vi "Read Version.vi"(8 "error in (no error)":errorcluster, 11 "Engine in":refnum<class "Engine.lvclass">) -> (0 "error out":errorcluster, 2 "Version":string, 3 "Engine out":refnum<class "Engine.lvclass">)   [LabVIEW 2023, in "Engine.lvlib" / "Engine.lvclass"]
uses:
  Library/Engine.lvclass
  Library/Engine.lvclass/Engine.ctl
  <vilib>/Utility/LVLibp/NI_PackedLibraryUtility.lvlib
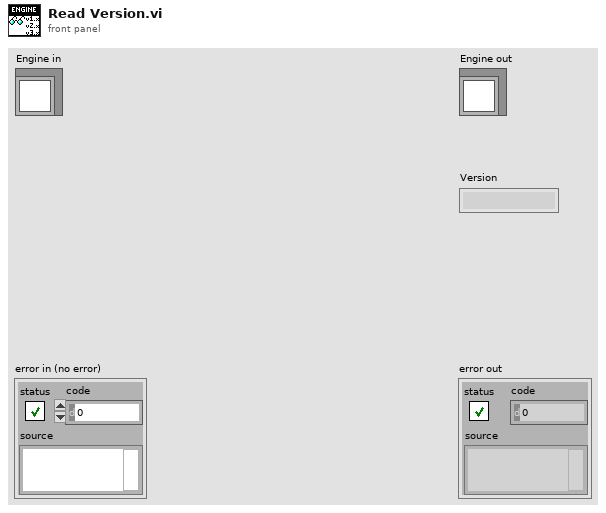
[diagram p1: front panel]
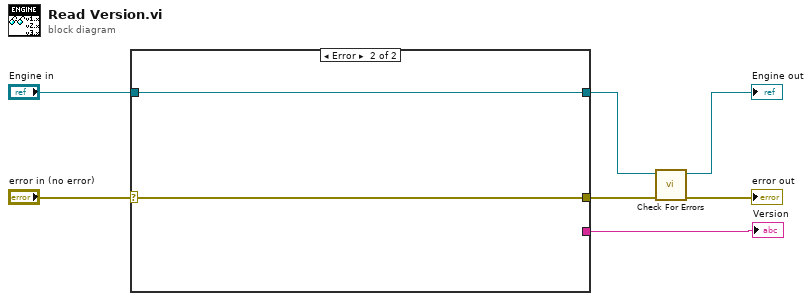
[diagram p0: block diagram]
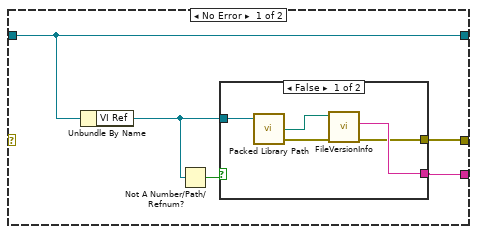
[diagram p2: hidden frame]
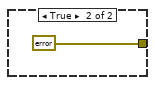
[diagram p3: hidden frame]
diagram:
  n1 = case shown="Error" "error in (no error)" {
    selector: "error in (no error)" -> [_ w20]
    tunnel: [w8 w20] -> w6
    tunnel: [w12 w19] -> w2
    tunnel: "Engine in" -> [w12 w19]
    tunnel: [w9 _] -> w4
    frame No Error {
      n2 = Unbundle By Name(w12) -> ("VI Ref"=w10:refnum<vi>)
      n3 = Not A Number/Path/Refnum?(number/path/refnum=w10) -> (NaN/Path/Refnum?=w11:bool)
      n4 = case shown="False" w11 {
        tunnel: [w15 _] -> w9
        tunnel: w10 -> [w17 _]
        tunnel: [w13 errorcluster {"status"=TRUE, "code"=7, "source"=""} ("error out")] -> w8
        frame False {
          n5 = call <vilib>:"Packed Library Path.vi"("vi reference"=w17) -> ("error out"=w14:errorcluster, "packed library path"=w16:path)  [unwired: 2 in, 1 out]
          n6 = call <vilib>:"FileVersionInfo.vi"("error in (no error)"=w14, "Application Path in"=w16) -> ("error out"=w13:errorcluster, "File Version Info"=w15:string)  [unwired: 6 in, 2 out]
        }
        frame True {
        }
      }
    }
    frame Error {
    }
  }
  "Version" <- w4
  n7 = call "Check For Errors.vi"("error in"=w6, "Engine in"=w2) -> ("error out"=→"error out":errorcluster, "Engine out"=→"Engine out":refnum<class "Engine.lvclass">)  [unwired: 8 in]
